vi "PathPlanner_CommandUtil_DoWait.vi"(9 "PassthroughTime_SEC":dbl=-1.0, 10 "Init":bool, 11 "WaitTimeSec":dbl) -> (3 "Done":bool)   [LabVIEW 2019, in "PathPlanner24.lvlib"]
uses:
  PathPlanner24.lvlib
  <vilib>/Utility/semaphor.llb/Obtain Semaphore Reference.vi
  <vilib>/Rock Robotics/WPI/ThirdParty/JAS_Junk/TrajLib/Timer_Reset.vi
  <vilib>/Rock Robotics/WPI/ThirdParty/JAS_Junk/TrajLib/Trajectory_Library.lvlib
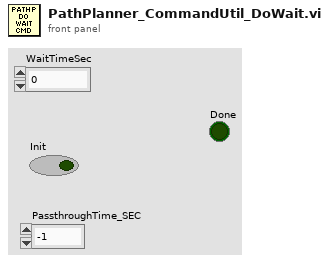
[diagram p1: front panel]
types:
  T1 = typedef "Trajectory_Library.lvlib/TIMER.ctl" = cluster{"StartTime":dbl, "Accumulated TIme":dbl, "Running":bool, "semaphore":T2}
  T2 = typedef "Semaphore RefNum" = refnum<k1>
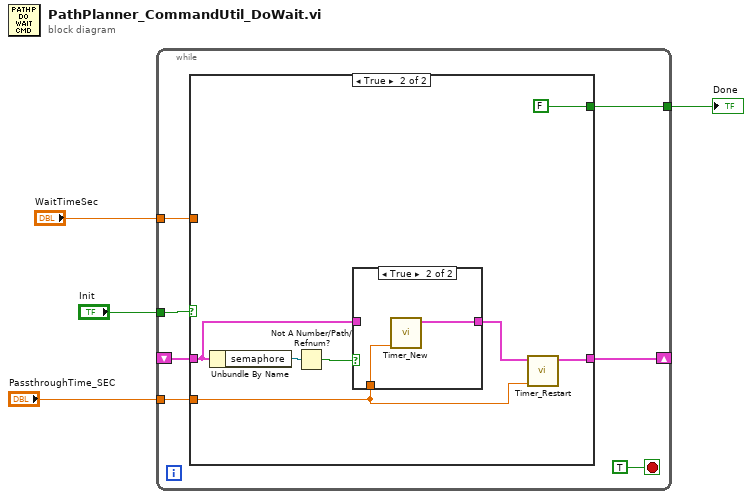
[diagram p0: block diagram]
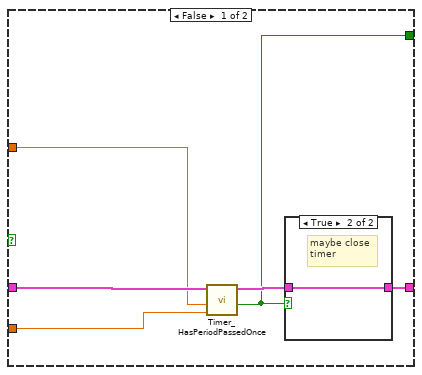
[diagram p2: hidden frame]
diagram:
  n1 = while {
    tunnel: "Init" -> [w11]
    tunnel: "PassthroughTime_SEC" -> [w10]
    shift-right: [w9] -> _
    shift-left: _ -> [w8]
    tunnel: [w6] -> w1
    tunnel: "WaitTimeSec" -> [w5]
    stop <- TRUE stop-if-true
    n2 = case shown="True" w11 {
      tunnel: w10 -> [w16 w25]
      tunnel: [w14 w24] -> w9
      tunnel: w8 -> [w17 w20]
      tunnel: [w13 FALSE ("Expired")] -> w6
      tunnel: w5 -> [w12 _]
      frame False {
        n3 = call <vilib>:"Timer_HasPeriodPassedOnce.vi"("Pass_Through_Time"=w16, "Period"=w12, "in Timer"=w17) -> ("Expired"=w13:bool, "out Timer"=w15:T1)  [unwired: 6 in, 1 out]
        n4 = case shown="True" w13 {
          tunnel: w15 -> [w18 w19]
          tunnel: [w18 w19] -> w14
          frame False {
          }
          frame True {
            # "maybe close\ntimer"
          }
        }
      }
      frame True {
        n5 = Unbundle By Name(w20) -> ("semaphore"=w21:T2)
        n6 = Not A Number/Path/Refnum?(number/path/refnum=w21) -> (NaN/Path/Refnum?=w22:bool)
        n7 = case shown="True" w22 {
          tunnel: [w27 w29] -> w26
          tunnel: w25 -> [_ w28]
          tunnel: w20 -> [w27 _]
          frame False {
          }
          frame True {
            n8 = call <vilib>:"Timer_New.vi"("Pass_Through_Time"=w28) -> ("TIMER"=w29:T1)  [unwired: 10 in]
          }
        }
        n9 = call <vilib>:"Timer_Restart.vi"("Pass_Through_Time"=w25, "in Timer"=w26) -> ("out Timer"=w24:T1)  [unwired: 9 in]
      }
    }
  }
  "Done" <- w1
